vi "slam3.vi"(7 "Xin":dbl[](array[numeric])=[0.0, 0.0, 0.0], 8 "error in":errorcluster, 9 "measurements":dbl[][](array[numeric]), 10 "dX":dbl[](array[numeric]), 11 "Pin":dbl[][](array[numeric])=[[0.01, 0.0, 0.0], [0.0, 0.01, 0.0], [0.0, 0.0, 0.01]]) -> (0 "error out":errorcluster, 1 "measuredLandmarks":dbl[][](array[numeric]), 2 "Xodometry":dbl[](array[numeric]), 3 "Pout":dbl[][](array[numeric]), 5 "Xout":dbl[](array[numeric]))   [LabVIEW 2009]
uses:
  Matlab/SLAM.m
  LabVIEW Data/MathScriptVIs/MCStatic_151019524_e1a397bcafc81a1fbed368d2c996ebff.vi
  Matlab/addLandmark.m
  Matlab/associateToLandmark.m
  Matlab/assOrAddLandmark.m
  Matlab/dist.m
  Matlab/distance.m
  Matlab/findRangeBearing.m
  Matlab/shiftAngle.m
  Matlab/updateFromLandmarks.m
  Matlab/updateFromOdometry.m
  <vilib>/imath/engines/lvmath2/RunTimeEngine/ErrorHandling/NIMS_Finalize Error.vi
  <vilib>/imath/engines/lvmath2/RunTimeEngine/Parser/MC_Version.vi
  <vilib>/imath/engines/lvmath2/RunTimeEngine/Managers/WorkSpace/UID Generator.vi
  <vilib>/imath/engines/lvmath2/RunTimeEngine/NodeEndStatement/NIMS_NodeEndStatement_Output.vi
  <instcachedir>/0/NIMS_NodeEndStatement_Output_B70DDD75627E4997AAE11E9955EDAA25.lvgen/NIMS_NodeEndStatement_Output_B70DDD75627E4997AAE11E9955EDAA25_008.vi
  <instcachedir>/0/NIMS_NodeEndStatement_Output_B70DDD75627E4997AAE11E9955EDAA25.lvgen/NIMS_NodeEndStatement_Output_B70DDD75627E4997AAE11E9955EDAA25_007.vi
  <instcachedir>/0/NIMS_NodeEndStatement_Output_B70DDD75627E4997AAE11E9955EDAA25.lvgen/NIMS_NodeEndStatement_Output_B70DDD75627E4997AAE11E9955EDAA25_005.vi
  <instcachedir>/0/NIMS_NodeEndStatement_Output_B70DDD75627E4997AAE11E9955EDAA25.lvgen/NIMS_NodeEndStatement_Output_B70DDD75627E4997AAE11E9955EDAA25_001.vi
  <vilib>/imath/engines/lvmath2/RunTimeEngine/Managers/SymbolTable/Clear UID.vi
  <vilib>/imath/engines/lvmath/Functions/Error Handling/MergeErrorsWrapper.vi
  <instcachedir>/0/MCStatic_151019524_e1a397bcafc81a1fbed368d2c996ebff_851D8408E3074C86B6B330D7E2AB0140.lvgen/MCStatic_151019524_e1a397bcafc81a1fbed368d2c996ebff_851D8408E3074C86B6B330D7E2AB0140_000.vi
  <vilib>/imath/engines/lvmath2/RunTimeEngine/Managers/SymbolTable/NIMS_WorkSpace.lvlib
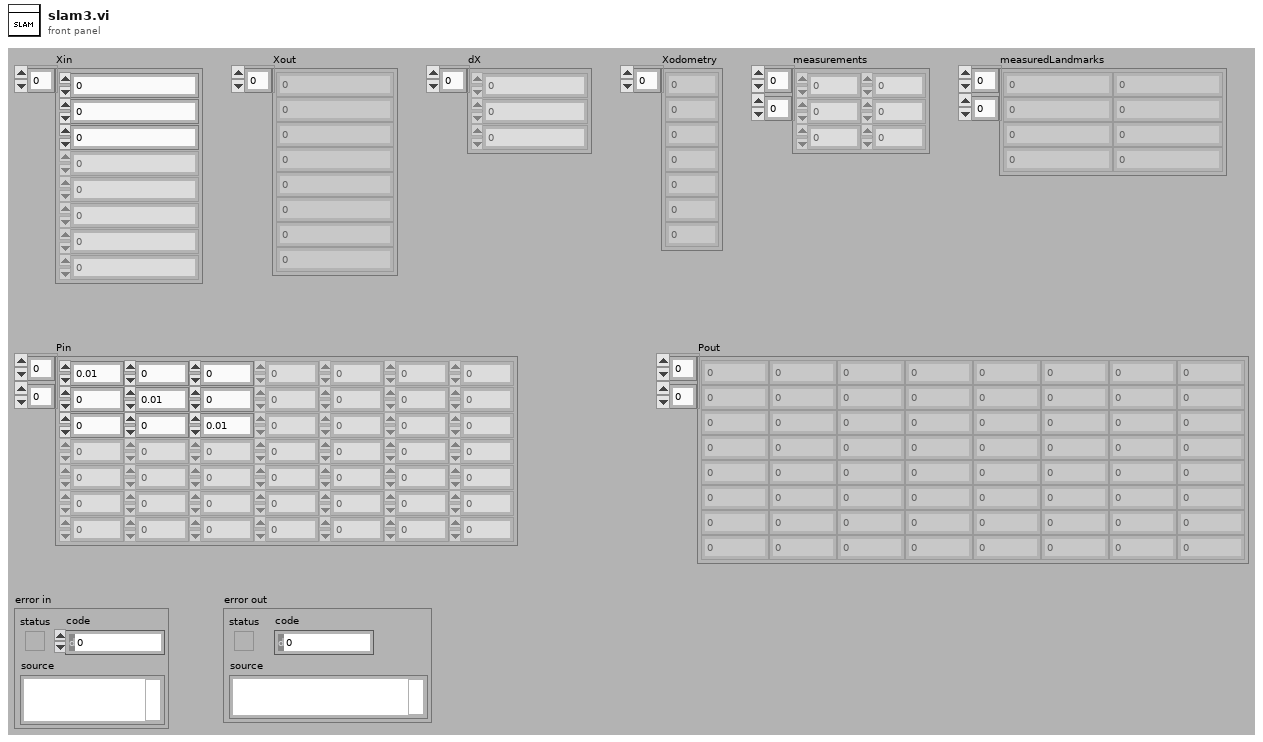
[diagram p1: front panel]
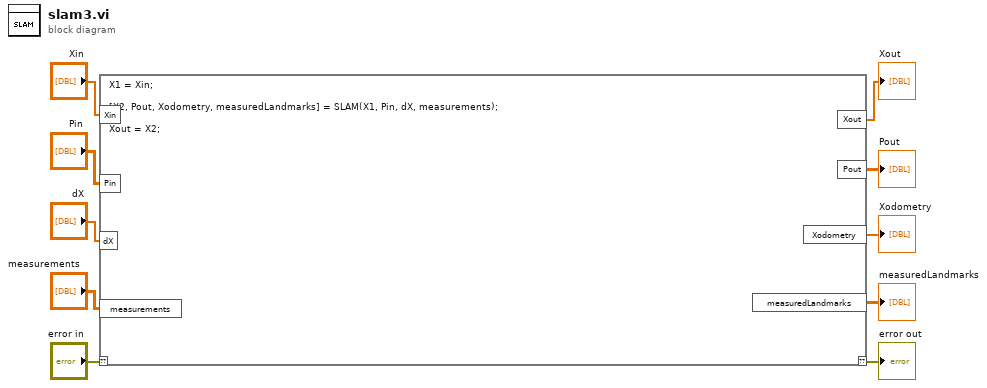
[diagram p0: block diagram]
diagram:
  n1 = mathscript code="X1 = Xin;\n  \n[X2, Pout, Xodometry, measuredLandmarks] = SLAM(X1, Pin, dX, measurements);\n\nXout = X2;"("??"="error in", "Xin"="Xin", "Pin"="Pin", "dX"="dX", "measurements"="measurements") -> ("??"=→"error out":errorcluster, "Xout"=→"Xout":cdb[], "Pout"=→"Pout":cdb[][], "Xodometry"=→"Xodometry":dbl[], "measuredLandmarks"=→"measuredLandmarks":dbl[][])
